vi "ButtonCheck.vi"(10 "Error In":errorcluster, 11 "Button Ref":refnum<vi>) -> (2 "error out":errorcluster, 3 "Enabled?":bool)   [LabVIEW 2015]
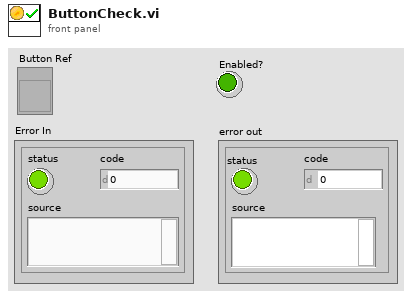
[diagram p1: front panel]
types:
  T1 = enum8{"Enabled", "Disabled", "Disabled and Grayed Out"}
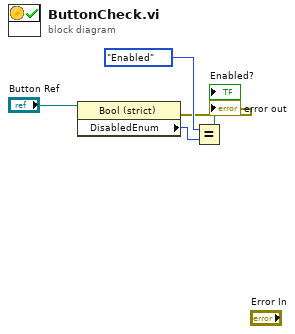
[diagram p0: block diagram]
diagram:
  n1 = property class="Bool (strict)"(reference="Button Ref") -> (error out=→"error out":errorcluster, "DisabledEnum"=w4:T1)  [unwired: 1 in, 1 out]
  n2 = Equal?(x=T1."Enabled" ("Disabled"), y=w4) -> (x = y?=→"Enabled?":bool)
